vi "host - network - RT (separate).vi"() -> ()   [LabVIEW 2021]
panel:
  in  "stop":bool
  out "data":dbl(graph)
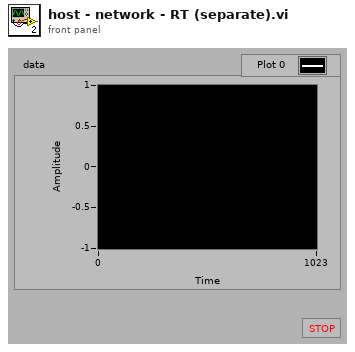
[diagram p1: front panel]
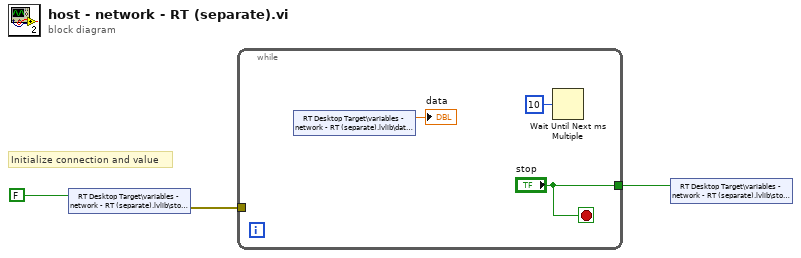
[diagram p0: block diagram]
diagram:
  # "Initialize connection and value"
  n1 = shared-variable "RT Desktop Target\\variables - network - RT (separate).lvlib\\stop - network"(FALSE) -> (error out=w2:errorcluster)  [unwired: 1 in]
  n2 = while {
    tunnel: ["stop"] -> w3
    tunnel: w2 -> [_]
    stop <- "stop" stop-if-true
    n3 = shared-variable "RT Desktop Target\\variables - network - RT (separate).lvlib\\data - network"() -> (→"data":dbl)  [unwired: 1 in, 1 out]
    n4 = Wait Until Next ms Multiple(millisecond multiple=u32 10) -> ()  [unwired: 1 out]
  }
  n5 = shared-variable "RT Desktop Target\\variables - network - RT (separate).lvlib\\stop - network"(w3) -> ()  [unwired: 1 in, 1 out]
